vi "PBI_MFA_Interface_DriveEnable2-Axis1.vi"() -> (0 "DriveEnableStatus":bool, 1 "DriveEnableError":bool)   [LabVIEW 2011]
panel:
  out "error AAABuild":errorcluster
  out "error SetUSBlink":errorcluster
  out "AAABuild 2":i32
  out "error DriveEnableOut":errorcluster
  out "error DriveEnableIn":errorcluster
  out "AAABuild":i32
  in  "MintController":refnum<k7>(container)
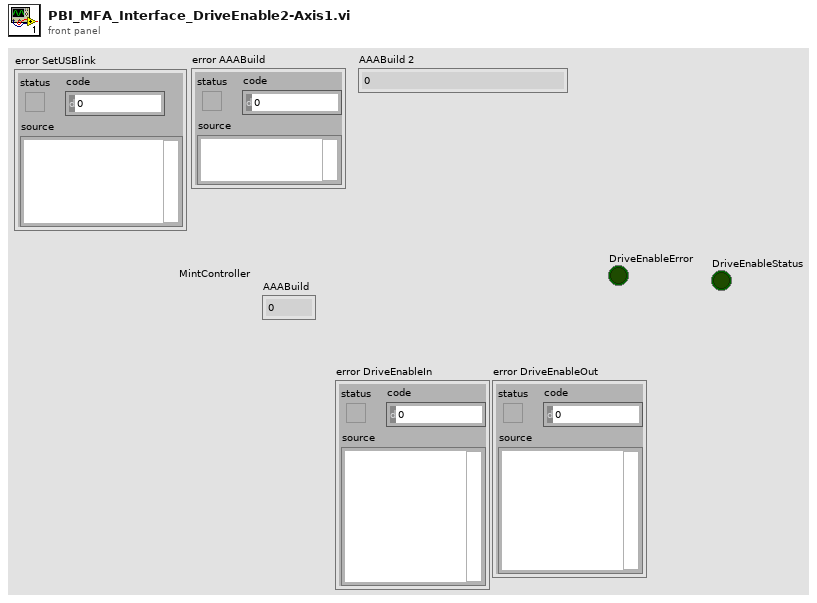
[diagram p1: front panel]
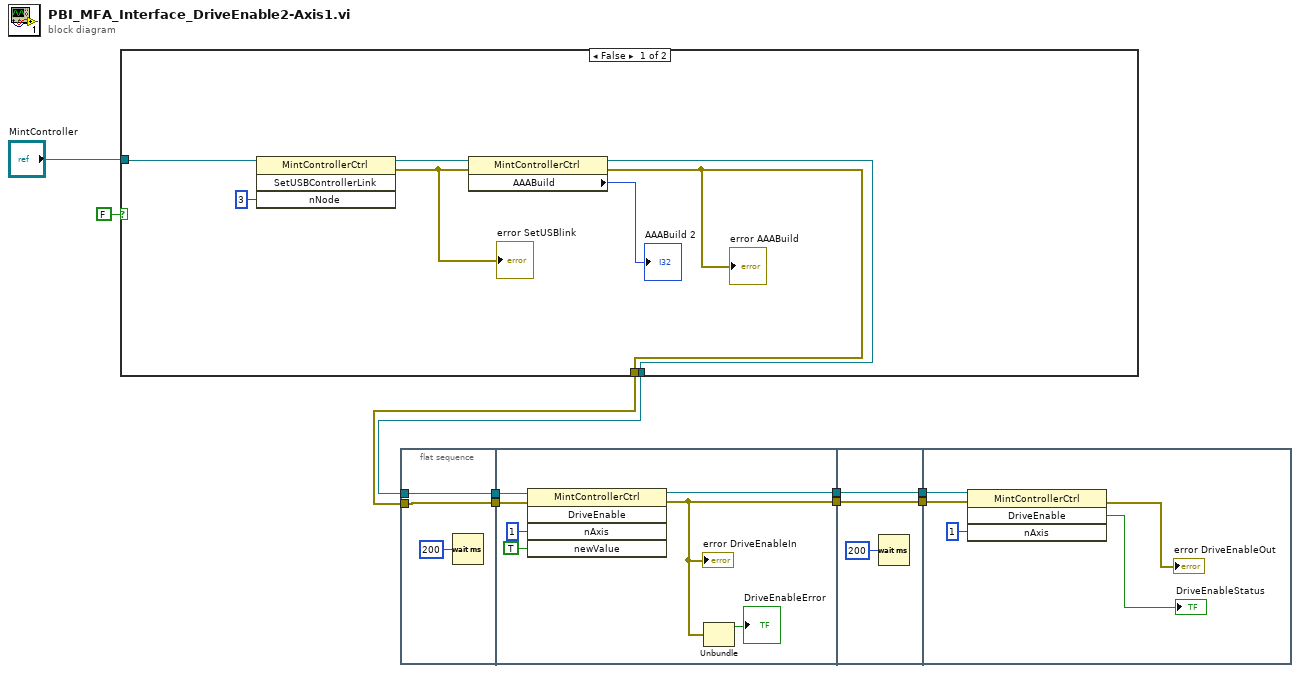
[diagram p0: block diagram]
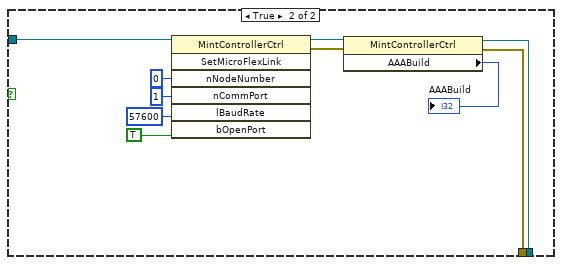
[diagram p2: hidden frame]
diagram:
  n1 = case shown="False" FALSE {
    tunnel: "MintController" -> [w13 w26]
    tunnel: [w12 w19] -> w5
    tunnel: [w11 w18] -> w4
    frame False {
      n2 = invoke class="MintControllerCtrl" method="SetUSBControllerLink"(reference=w13, "nNode"=i16 3) -> (reference out=w15:refnum<k7>, error out=w14:errorcluster)  [unwired: 2 in, 2 out]
      "error SetUSBlink" <- w14
      n3 = property class="MintControllerCtrl"(reference=w15, error in=w14) -> (reference out=w12:refnum<k7>, error out=w11:errorcluster, "AAABuild"=→"AAABuild 2":i32)
      "error AAABuild" <- w11
    }
    frame True {
      n4 = invoke class="MintControllerCtrl" method="SetMicroFlexLink"(reference=w26, "nNodeNumber"=i16 0, "nCommPort"=i16 1, "lBaudRate"=57600, "bOpenPort"=TRUE) -> (reference out=w27:refnum<k7>, error out=w21:errorcluster)  [unwired: 2 in, 5 out]
      n5 = property class="MintControllerCtrl"(reference=w27, error in=w21) -> (reference out=w19:refnum<k7>, error out=w18:errorcluster, "AAABuild"=→"AAABuild":i32)
    }
  }
  n6 = flat-sequence {
    tunnel: w5 -> [w29]
    tunnel: [w29] -> w2
    tunnel: w4 -> [w28]
    tunnel: [w28] -> w1
    tunnel: [w31] -> w8
    tunnel: [w33] -> w6
    tunnel: w2 -> [w37]
    tunnel: w1 -> [w36]
    tunnel: [w39] -> w9
    tunnel: w8 -> [w39]
    tunnel: [w38] -> w7
    tunnel: w6 -> [w38]
    tunnel: w9 -> [w44]
    tunnel: w7 -> [w45]
    frame #0 {
      n7 = Wait (ms)(milliseconds to wait=u32 200) -> ()  [unwired: 1 out]
    }
    frame #1 {
      n8 = invoke class="MintControllerCtrl" method="DriveEnable"(reference=w37, error in=w36, "nAxis"=i16 1, "newValue"=TRUE) -> (reference out=w33:refnum<k7>, error out=w31:errorcluster)  [unwired: 1 in, 3 out]
      "error DriveEnableIn" <- w31
      n9 = Unbundle(w31) -> ("status"=→"DriveEnableError":bool)  [unwired: 2 out]
    }
    frame #2 {
      n10 = Wait (ms)(milliseconds to wait=u32 200) -> ()  [unwired: 1 out]
    }
    frame #3 {
      n11 = invoke class="MintControllerCtrl" method="DriveEnable"(reference=w45, error in=w44, "nAxis"=i16 1) -> (error out=→"error DriveEnableOut":errorcluster, "DriveEnable"=→"DriveEnableStatus":bool)  [unwired: 1 in, 2 out]
    }
  }
